vi "Read PrechargeTimeout.vi"(8 "error in (no error)":errorcluster, 11 "AppStateMachine configuration in":refnum<class "AppStateMachine configuration.lvclass">) -> (0 "error out":errorcluster, 2 "PrechargeTimeout":u32, 3 "AppStateMachine configuration out":refnum<class "AppStateMachine configuration.lvclass">)   [LabVIEW 2017, in "AppStateMachine configuration.lvclass"]
uses:
  AppStateMachine configuration.lvclass
  AppStateMachine configuration.lvclass/AppStateMachine configuration.ctl
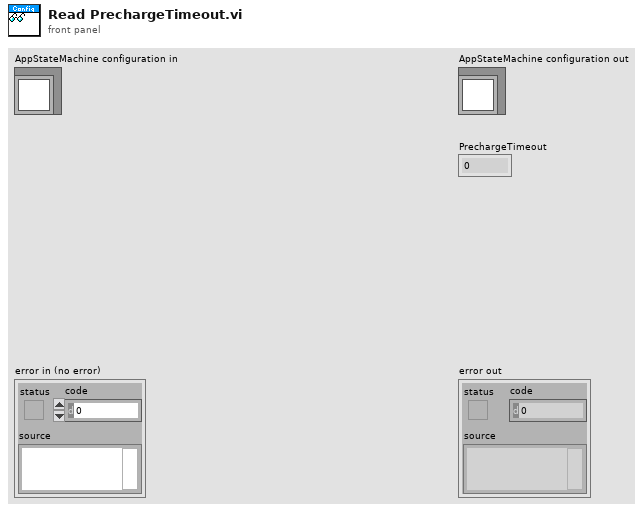
[diagram p1: front panel]
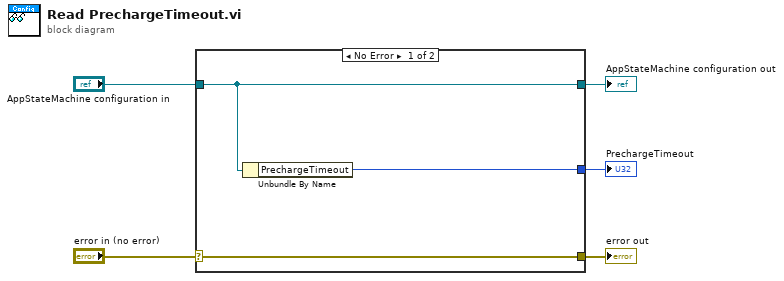
[diagram p0: block diagram]
diagram:
  n1 = case shown="No Error" "error in (no error)" {
    selector: "error in (no error)" -> [w8 w9]
    tunnel: [w8 w9] -> w4
    tunnel: [w7 w10] -> w2
    tunnel: "AppStateMachine configuration in" -> [w7 w10]
    tunnel: [w6 _] -> w1
    frame No Error {
      n2 = Unbundle By Name(w7) -> ("PrechargeTimeout"=w6:u32)
    }
    frame Error {
    }
  }
  "error out" <- w4
  "AppStateMachine configuration out" <- w2
  "PrechargeTimeout" <- w1
